vi "Evaluate Derivative.vi"(1 "x":dbl, 3 "Function Reference":refnum<vi>) -> (0 "f'(x)":dbl)   [LabVIEW 2020, in "Automatic Differentiation.lvlib"]
uses:
  Automatic Differentiation.lvlib
  classes/Dual/Dual.lvclass
  classes/Dual/Dual.lvclass/Dual.ctl
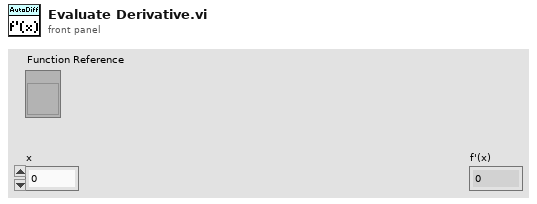
[diagram p1: front panel]
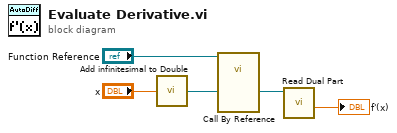
[diagram p0: block diagram]
diagram:
  n1 = call "Add infinitesimal to Double.vi"("DBL (x)"="x") -> ("Dual (x+e)"=w3:refnum<class "Dual.lvclass">)
  n2 = call-by-ref "?"(reference="Function Reference", "x"=w3) -> ("f(x)"=w2:refnum<class "Dual.lvclass">)  [unwired: 1 in, 2 out]
  n3 = call "Read Dual Part.vi"("Dual in"=w2) -> ("Dual Part"=→"f'(x)":dbl)  [unwired: 9 in, 1 out]
